vi "NoDynamicIOref.vi"() -> ()   [LabVIEW 2014]
uses:
  <vilib>/eio/EIONode/EIONode.xnode
  <vilib>/rvi/eio/common/nirviEmuTemplateMethod_errors.vi
panel:
  in  "index":i32
  out "I/O Item":i16
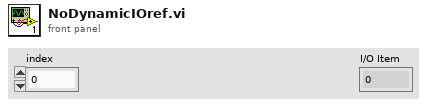
[diagram p1: front panel]
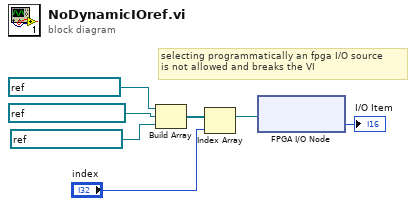
[diagram p0: block diagram]
diagram:
  # "selecting programmatically an fpga I/O source\nis not allowed and breaks the VI"
  n1 = Build Array(refnum<k21> "Connector0/AI0" ("FPGA I/O In"), refnum<k21> "Connector0/AI1" ("FPGA I/O In"), refnum<k21> "Connector0/AI2" ("FPGA I/O In")) -> (w4:refnum<k21>[])
  n2 = Index Array(array=w4, index="index") -> (element=w3:refnum<k21>)
  n3 = xnode "FPGA I/O Node"("FPGA I/O In"=w3) -> ("I/O Item"=→"I/O Item":i16)  [unwired: 1 out]
